vi "our rocket league.vi"(11 "Axes":dbl[](array[numeric])) -> (1 "upper limit":dbl, 2 "upper limit 2":dbl, 3 "upper limit 3":dbl)   [LabVIEW 2019]
uses:
  <vilib>/Rock Robotics/Network Tables/NT Read String.vi
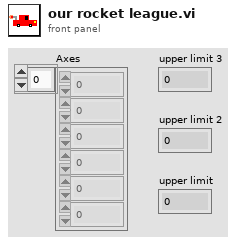
[diagram p1: front panel]
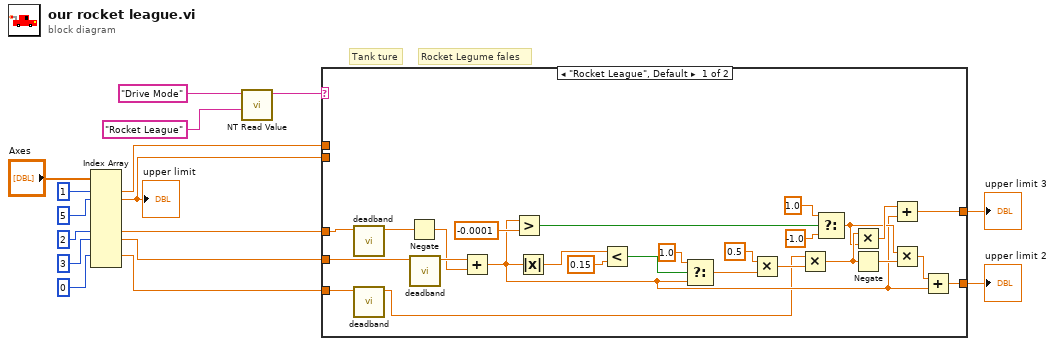
[diagram p0: block diagram]
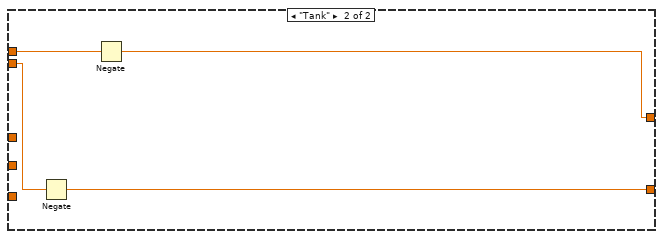
[diagram p2: hidden frame]
diagram:
  # "Rocket Legume fales"
  # "Tank ture"
  n1 = Index Array(array="Axes", index #1=1 ("index"), index #2=5 ("index"), index #6=2 ("index"), index #7=3 ("index"), index #9=0 ("index")) -> (element #1=w4:dbl, element #2=w16:dbl, element #6=w9:dbl, element #7=w10:dbl, element #9=w15:dbl)  [unwired: 5 in, 5 out]
  "upper limit" <- w16
  n2 = call-poly <vilib>:"NT Read Value.vi"("Default Value"="Rocket League", "Name"="Drive Mode") -> ("String"=w12:string)  [unwired: 8 in, 1 out]
  n3 = case shown="\"Rocket League\", Default" w12 {
    tunnel: w4 -> [_ w46]
    tunnel: w16 -> [_ w44]
    tunnel: [w27 w45] -> w5
    tunnel: [w28 w43] -> w6
    tunnel: w9 -> [w25 _]
    tunnel: w10 -> [w26 _]
    tunnel: w15 -> [w24 _]
    frame "Rocket League", Default {
      n4 = call "deadband.vi"("Joystick Value"=w25) -> ("Val"=w42:dbl)  [unwired: 10 in]
      n5 = call "deadband.vi"("Joystick Value"=w24) -> ("Val"=w17:dbl)  [unwired: 10 in]
      n6 = Negate(x=w42) -> (-x=w40:dbl)
      n7 = call "deadband.vi"("Joystick Value"=w26) -> ("Val"=w41:dbl)  [unwired: 10 in]
      n8 = Add(x=w41, y=w40) -> (x+y=w22:dbl)
      n9 = Greater?(x=w22, y=-0.0001) -> (0:w38:bool)
      n10 = Absolute Value(x=w22) -> (abs(x)=w21:dbl)
      n11 = Less?(x=w21, y=0.15) -> (x < y?=w19:bool)
      n12 = Select(t=1.0, s=w19, f=w22) -> (s? t:f=w18:dbl)
      n13 = Multiply(x=0.5, y=w18) -> (x*y=w30:dbl)
      n14 = Multiply(x=w17, y=w30) -> (x*y=w35:dbl)
      n15 = Select(t=1.0, s=w38, f=-1.0) -> (s? t:f=w33:dbl)
      n16 = Multiply(x=w35, y=w33) -> (x*y=w34:dbl)
      n17 = Negate(x=w35) -> (-x=w32:dbl)
      n18 = Add(x=w34, y=w22) -> (x+y=w27:dbl)
      n19 = Multiply(x=w33, y=w32) -> (x*y=w31:dbl)
      n20 = Add(x=w31, y=w22) -> (x+y=w28:dbl)
    }
    frame "Tank" {
      n21 = Negate(x=w44) -> (-x=w43:dbl)
      n22 = Negate(x=w46) -> (-x=w45:dbl)
    }
  }
  "upper limit 2" <- w6
  "upper limit 3" <- w5
